vi "Versioned Load.vi"(10 "path":path) -> (0 "Reversals":T10, 1 "Trajectory Data":T1, 2 "Zero V":bool, 3 "Commands out":cluster{"Time (s)":dbl, T8, bool}[](array[cluster]), 4 "Fields":T7 {"Overrides"."Angle Override" step=5.0; "Overrides"."Velocity Override" step=5.0; "Overrides"."Angular Override" step=5.0; "Angular Limits"."Jerk (deg/s^3)" min=0.0 step=1.0; "Angular Limits"."Accel (deg/s^2)" min=0.0; "Angular Limits"."Velocity (deg/s)" min=0.0}, 5 "Points out":cluster{"x":dbl, "y":dbl, "th":dbl}[](array[cluster]), 6 "Trajectory Meta":cluster{"Drive Type":T3, "Path Type":T4}, 7 "Overall":cluster{"Time (s)":dbl, "Distance (ft)":dbl}, 8 "error out":errorcluster)   [LabVIEW 2023]
uses:
  Types/Single Cmd Info.ctl
  <vilib>/picture/picture.llb/imagedata.ctl
  Types/Overrides.ctl
  Types/Angluar Limits.ctl
  Types/Drive Type.ctl
  Types/Path Type.ctl
  Types/Trajectory Data.ctl
  Types/Segment Type.ctl
  Types/Availible Command systems for auto.ctl
  Types/Limits.ctl
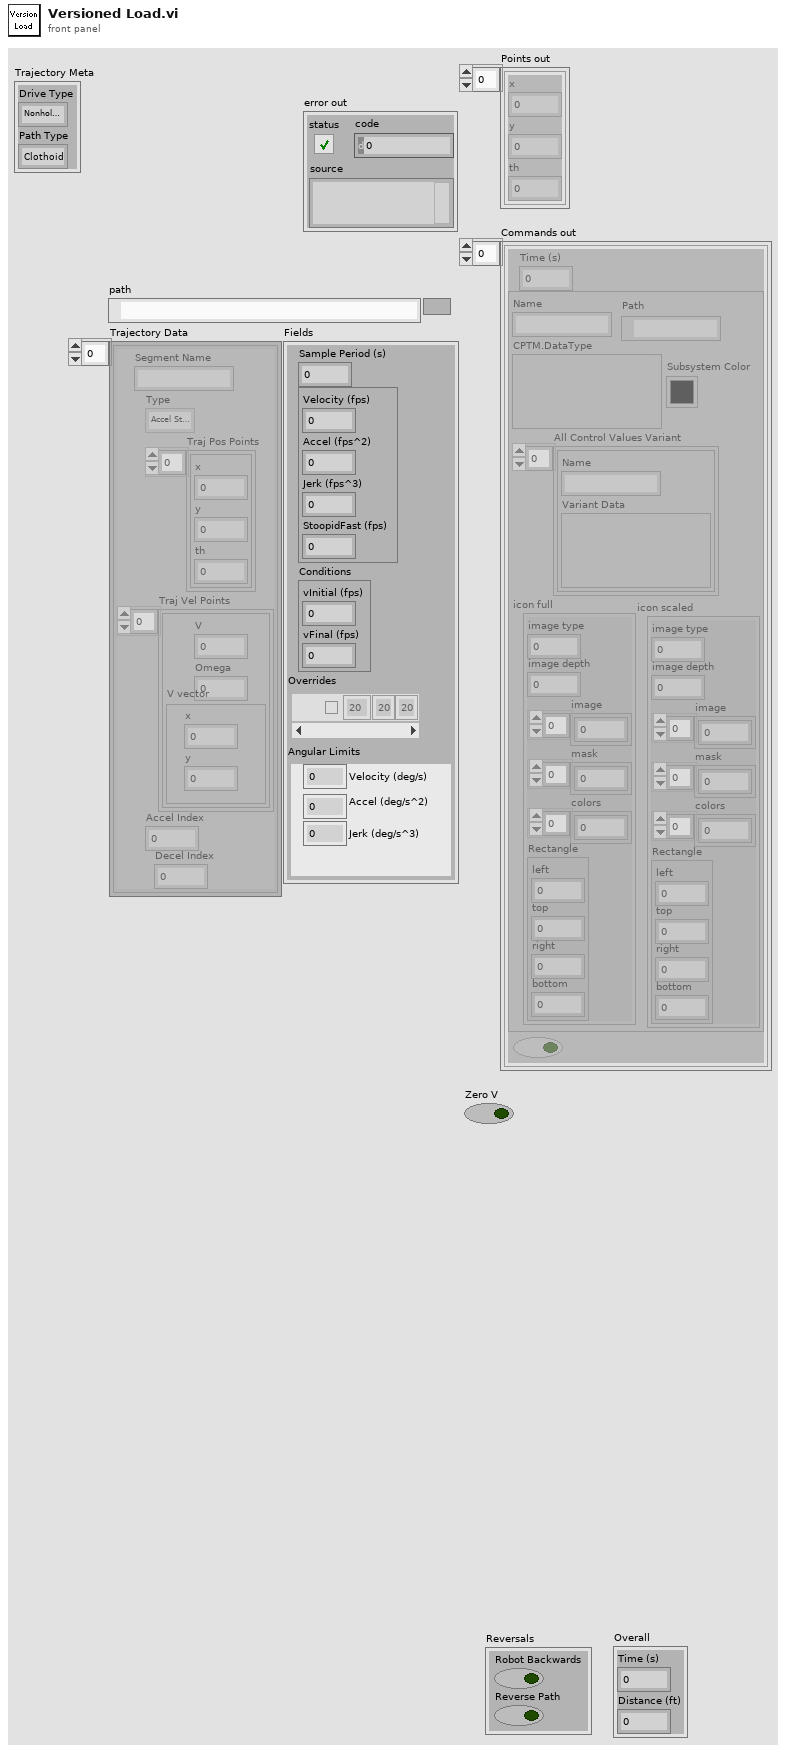
[diagram p1: front panel]
types:
  T1 = typedef "Trajectory Data.ctl" = cluster{"Segment Name":string, "Type":T2, "Traj Pos Points":cluster{"x":dbl, "y":dbl, "th":dbl}[], "Traj Vel Points":cluster{"V":dbl, "Omega":dbl, "V vector":cluster{"y":dbl, "x":dbl}}[], "Accel Index":i32, "Decel Index":i32}[]
  T2 = typedef "Segment Type.ctl" = enum16{"Accel Straight", "Const Straight", "Blend", "Circle", "Bezier"}
  T3 = typedef "Drive Type.ctl" = enum16{"Nonholonomic", "Holonomic"}
  T4 = typedef "Path Type.ctl" = enum16{"Clothoid", "Bezier"}
  T5 = typedef "Overrides.ctl" = cluster{"Count":string, "Angular Override":dbl, "Enabled?":bool, "Velocity Override":dbl, "Angle Override":dbl}[]
  T6 = typedef "Angluar Limits.ctl" = cluster{"Velocity (deg/s)":dbl, "Accel (deg/s^2)":dbl, "Jerk (deg/s^3)":dbl}
  T7 = cluster{"Sample Period (s)":dbl, cluster{"Velocity (fps)":dbl, "Accel (fps^2)":dbl, "Jerk (fps^3)":dbl, "StoopidFast (fps)":dbl}, "Conditions":cluster{"vInitial (fps)":dbl, "vFinal (fps)":dbl}, "Overrides":T5, "Angular Limits":T6}
  T8 = typedef "Single Cmd Info.ctl" = cluster{"Name":string, "CPTM.DataType":variant, "All Control Values Variant":cluster{"Name":string, "Variant Data":variant}[], "icon full":T9, "icon scaled":T9, "Path":path, "Subsystem Color":u32}
  T9 = typedef "imagedata.ctl" = cluster{"image type":i32, "image depth":i32, "image":u8[], "mask":u8[], "colors":u32[], "Rectangle":cluster{"left":i16, "top":i16, "right":i16, "bottom":i16}}
  T10 = cluster{"Robot Backwards":bool, "Reverse Path":bool}
  T11 = cluster{"Segment Name":string, "Type":T2, "Traj Pos Points":cluster{"x":dbl, "y":dbl, "th":dbl}[], "Traj Vel Points":cluster{"V":dbl, "Omega":dbl}[], "Accel Index":i32, "Decel Index":i32}[]
  T12 = cluster{"Sample Period (s)":dbl, "Limits 2":cluster{"Velocity (fps)":dbl, "Acceleration (fps^2)":dbl, "Jerk (fps^3)":dbl}, "Conditions":cluster{"vInitial (fps)":dbl, "vFinal (fps)":dbl}, " Acceleration Overrides":cluster{"Angular \nAccelerations":dbl[], "Accel Override Bools":bool[]}}
  T13 = cluster{"Velocity":dbl, "Sample Time":dbl, "Accel":dbl}
  T14 = cluster{"Sample Period (s)":dbl, "Limits":cluster{"Velocity (fps)":dbl, "Acceleration (fps^2)":dbl, "Jerk (fps^3)":dbl}, "Conditions":cluster{"vInitial (fps)":dbl, "vFinal (fps)":dbl}}
  T15 = cluster{"Sample Period (s)":dbl, "Limits":cluster{"Velocity (fps)":dbl, "Acceleration (fps^2)":dbl, "Jerk (fps^3)":dbl}, "Conditions":cluster{"vInitial (fps)":dbl, "vFinal (fps)":dbl}, "Min Rads":dbl[]}
  T16 = typedef "Availible Command systems for auto.ctl" = u16
  T17 = cluster{"Time into Path":dbl, "System":T16, "Item Selected?":bool, "System Selection":T16}[]
  T18 = cluster{"Sample Period (s)":dbl, "Limits 2":cluster{"Velocity (fps)":dbl, "Acceleration (fps^2)":dbl, "Jerk (fps^3)":dbl, "Stoopid Fast":dbl}, "Conditions":cluster{"vInitial (fps)":dbl, "vFinal (fps)":dbl}, " Acceleration Overrides":cluster{"Angular \nAccelerations":dbl[], "Accel Override Bools":bool[]}}
  T19 = cluster{"Sample Period (s)":dbl, "Limits":cluster{"Velocity (fps)":dbl, "Accel (fps^2)":dbl, "Turn Accel (fps^2)":dbl, "Jerk (fps^3)":dbl}, "Conditions":cluster{"vInitial (fps)":dbl, "vFinal (fps)":dbl}, cluster{dbl[], bool[]}}
  T20 = cluster{"Reverse Path":bool, "Robot Backwards":bool}
  T21 = typedef "Limits.ctl" = cluster{"Velocity (fps)":dbl, "Accel (fps^2)":dbl, "Jerk (fps^3)":dbl, "StoopidFast (fps)":dbl}
  T22 = cluster{"Sample Period (s)":dbl, "Limits":T21, "Conditions":cluster{"vInitial (fps)":dbl, "vFinal (fps)":dbl}, "Overrides":T5, "Angular Limits":T6}
  T23 = cluster{"Velocity":dbl, "Accel":dbl, "Accel":dbl, "Velocity":dbl}
  T24 = cluster{"Velocity (fps)":dbl, "Acceleration (fps^2)":dbl, "Jerk (fps^3)":dbl}
  T25 = cluster{"vInitial (fps)":dbl, "vFinal (fps)":dbl}
  T26 = cluster{"Velocity (fps)":dbl, "Acceleration (fps^2)":dbl, "Jerk (fps^3)":dbl, "Velocity (fps)":dbl}
  T27 = cluster{string, "Angular Multiplier":dbl, bool, "Velocity (fps)":dbl, "Velocity (fps)":dbl}
  T28 = cluster{"Angular \nAccelerations":dbl[], "Accel Override Bools":bool[]}
  T29 = cluster{"Velocity (fps)":dbl, "Acceleration (fps^2)":dbl, "Jerk (fps^3)":dbl, "Stoopid Fast":dbl}
  T30 = cluster{"Velocity (fps)":dbl, "Accel (fps^2)":dbl, "Turn Accel (fps^2)":dbl, "Jerk (fps^3)":dbl}
  T31 = cluster{"Velocity (fps)":dbl, "Accel (fps^2)":dbl, "Jerk (fps^3)":dbl, "StoopidFast (fps)":dbl}
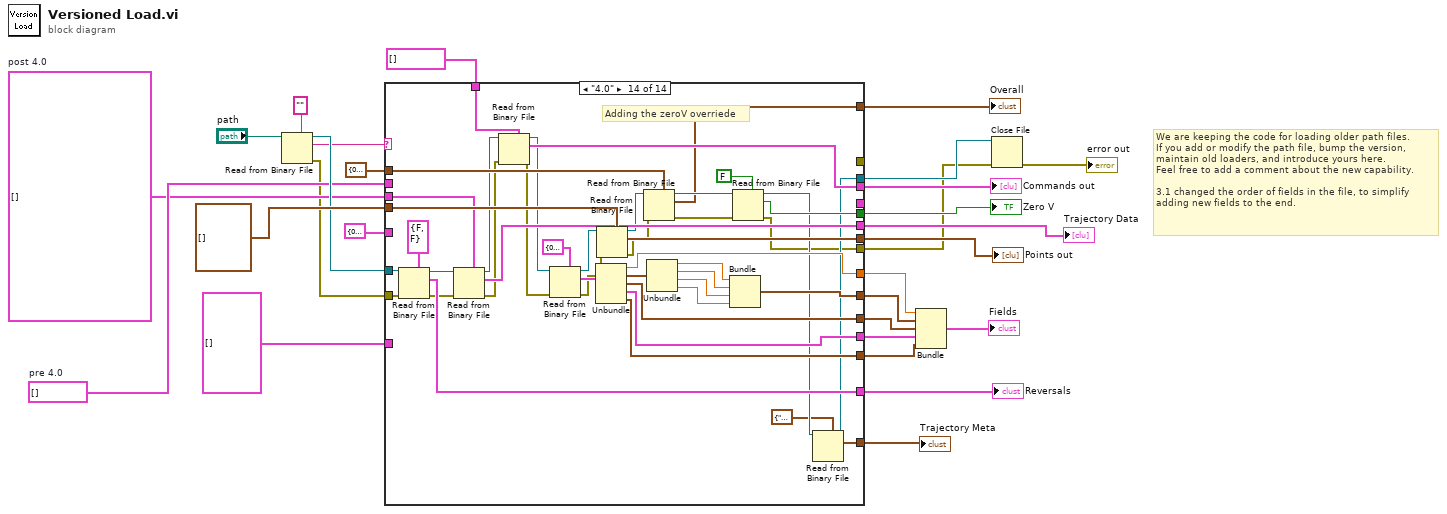
[diagram p0: block diagram]
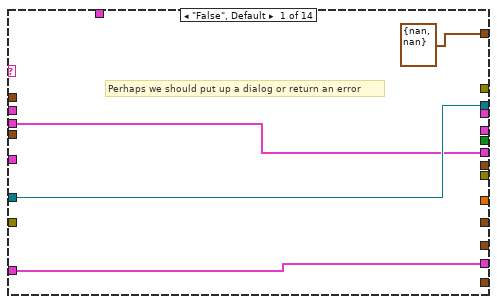
[diagram p2: hidden frame]
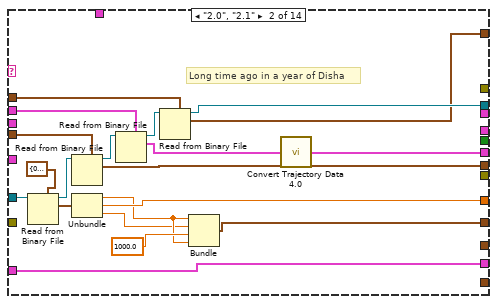
[diagram p3: hidden frame]
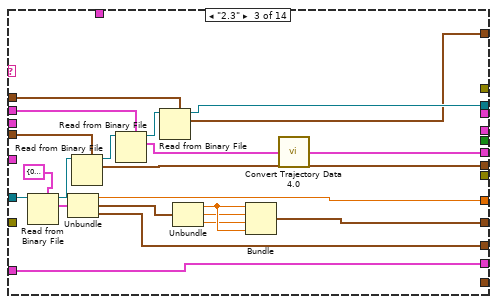
[diagram p4: hidden frame]
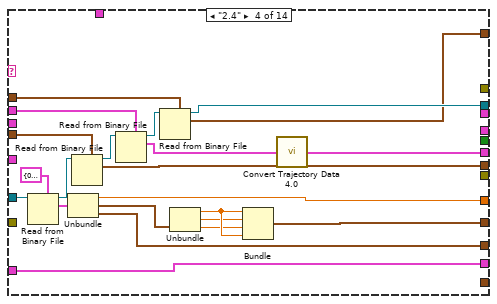
[diagram p5: hidden frame]
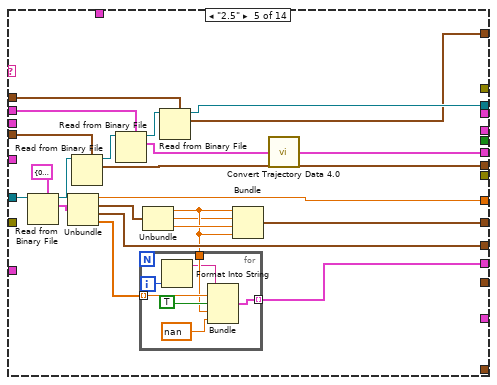
[diagram p6: hidden frame]
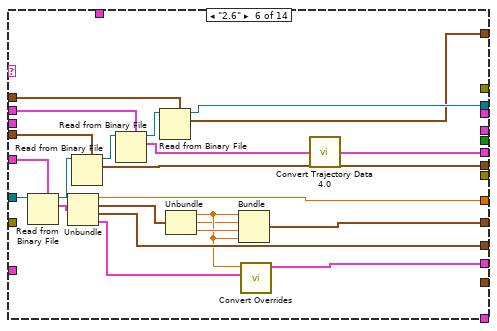
[diagram p7: hidden frame]
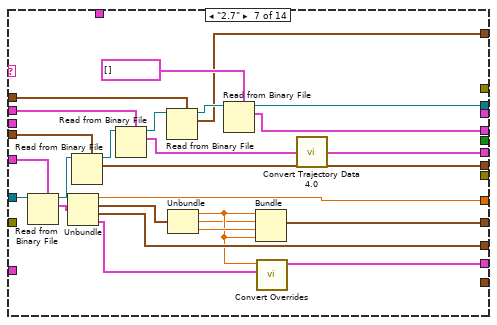
[diagram p8: hidden frame]
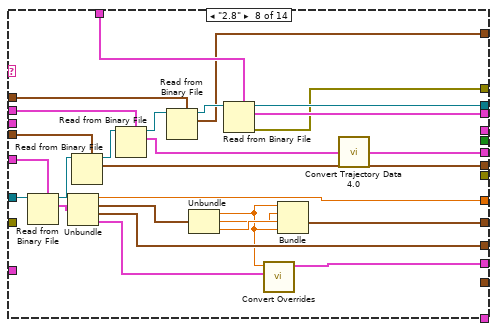
[diagram p9: hidden frame]
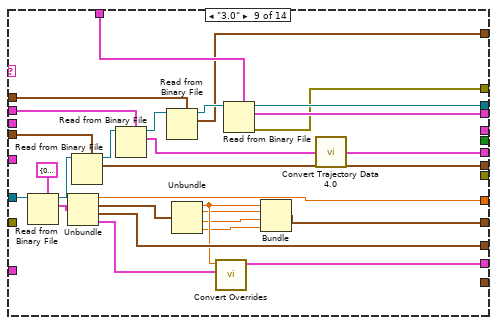
[diagram p10: hidden frame]
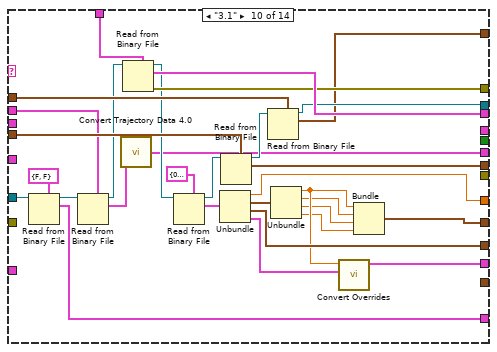
[diagram p11: hidden frame]
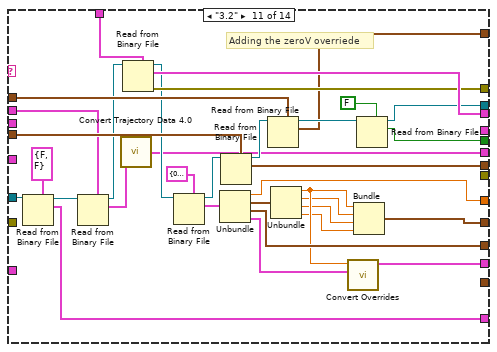
[diagram p12: hidden frame]
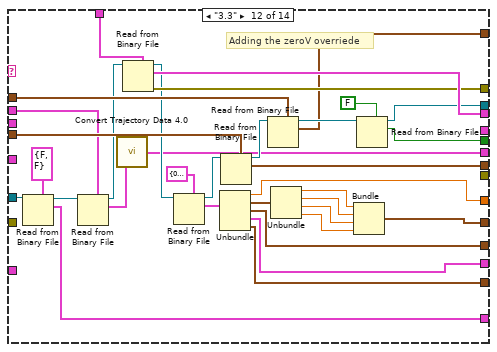
[diagram p13: hidden frame]
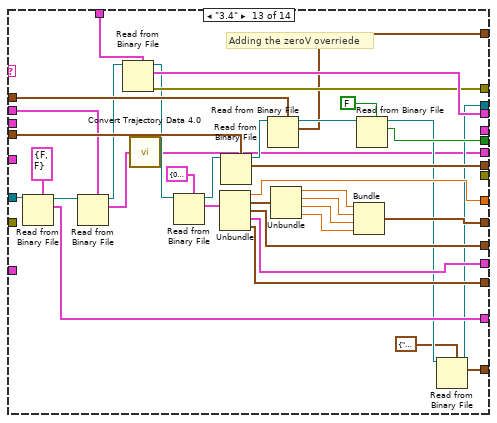
[diagram p14: hidden frame]
diagram:
  w6 = T11 []  # pre 4.0
  w5 = T1 []  # post 4.0
  # "We are keeping the code for loading older path files.\nIf you add or modify the path file, bump the version,\nmaintain old loaders, and introduce yours here.\nFeel free to add a comment about the new capability.\n\n3.1 changed the order of fields in the file, to simplify\nadding new fields to the end."
  n1 = Read from Binary File(5:"" ("String"), 11:"path") -> (0:w3:errorcluster, 2:w12:string, 3:w13:refnum<file>)  [unwired: 4 in, 1 out]
  n2 = case shown="\"4.0\"" w12 {
    tunnel: w13 -> [w32 w51 w73 w95 w118 w148 w174 w201 w229 w250 w284 w318 w355 w400]
    tunnel: cluster{"x":dbl, "y":dbl, "th":dbl}[] [] ("Points in") -> [_ w49 w71 w93 w116 w146 w172 w199 w227 w259 w293 w327 w364 w407]
    tunnel: [_ w48 w70 w92 w115 w145 w171 w198 w226 w258 w292 w326 w363 w406] -> w18
    tunnel: w6 -> [_ w47 w69 w91 w114 w144 w170 w197 w225 w257 w291 w325 w362 _]
    tunnel: cluster{"Time (s)":dbl, "Distance (ft)":dbl} {"Time (s)"=0.0, "Distance (ft)"=0.0} ("Cluster 4") -> [_ w45 w67 w89 w112 w142 w168 w195 w223 w256 w290 w324 w361 w405]
    tunnel: [w32 w43 w65 w87 w110 w140 w162 w189 w217 w246 w266 w303 w332 w377] -> w15
    tunnel: [_ w41 w64 w86 w109 w139 w166 w193 w221 w233 w268 w305 w342 w387] -> w25
    tunnel: [_ w37 w58 w79 w103 w134 w156 w184 w205 w238 w273 w310 w347 w392] -> w26
    tunnel: [_ _ w63 w85 w108 w138 w165 w192 w220 w255 w289 w323 w360 w404] -> w27
    tunnel: [w31 w36 w57 w78 w102 w132 w153 w181 w211 w242 w277 w298 w336 w381] -> w28
    tunnel: [w29 w33 w53 w75 w97 w127 w150 w176 w203 w231 w262 w296 w330 w403] -> w4
    tunnel: [_ _ _ _ _ _ w161 _ _ _ _ _ _ _] -> _
    tunnel: cluster{"Time (s)":dbl, T8, bool}[] [] ("Commands in") -> [_ _ _ _ _ _ _ w188 w216 w253 w287 w321 w358 w402]
    tunnel: [_ _ _ _ _ _ _ w187 w215 w252 w286 w320 w357 w401] -> w20
    tunnel: [_ _ _ _ _ _ _ w186 w214 w251 w285 w319 w356 _] -> _
    tunnel: T12 {"Sample Period (s)"=0.0, "Limits 2"={"Velocity (fps)"=0.0, "Acceleration (fps^2)"=0.0, "Jerk (fps^3)"=0.0}, "Conditions"={"vInitial (fps)"=0.0, "vFinal (fps)"=0.0}, " Acceleration Overrides"={"Angular \nAccelerations"=[], "Accel Override Bools"=[]}} ("Cluster") -> [_ _ _ _ _ w136 w159 w182 _ _ _ _ _ _]
    tunnel: [_ _ _ _ _ _ _ _ _ w241 w276 w312 w349 w394] -> w22
    tunnel: T5 [] ("Overrides") -> [w31 w36 w57 w78 _ _ _ _ _ _ _ _ _ _]
    tunnel: [_ _ _ _ _ _ _ _ _ _ w264 w301 w339 w384] -> w23
    tunnel: [cluster{"Time (s)":dbl, "Distance (ft)":dbl} {"Time (s)"=nan, "Distance (ft)"=nan} ("Cluster 4") w34 w54 w76 w98 w128 w151 w177 w204 w232 w263 w300 w338 w383] -> w10
    tunnel: [_ _ _ _ _ _ _ _ _ _ _ w297 w335 w380] -> w8
    tunnel: [_ _ _ _ _ _ _ _ _ _ _ _ w331 w376] -> w7
    tunnel: w5 -> [w29 _ _ _ _ _ _ _ _ _ _ _ _ w375]
    tunnel: w3 -> [_ _ _ _ _ _ _ _ _ _ _ _ _ w373]
    tunnel: [_ _ _ _ _ _ _ _ _ _ _ _ _ w367] -> w1
    frame "False", Default {
      # "Perhaps we should put up a dialog or return an error"
    }
    frame "2.0", "2.1" {
      # "Long time ago in a year of Disha"
      n3 = Read from Binary File(5:T13 {"Velocity"=0.0, "Sample Time"=0.0, "Accel"=0.0}, 11:w51) -> (2:w52:T13, 3:w50:refnum<file>)  [unwired: 4 in, 2 out]
      n4 = Read from Binary File(5:w49, 11:w50) -> (2:w48:cluster{"x":dbl, "y":dbl, "th":dbl}[], 3:w46:refnum<file>)  [unwired: 4 in, 2 out]
      n5 = Unbundle(w52) -> ("Velocity"=w38:dbl, "Sample Time"=w41:dbl, "Accel"=w35:dbl)
      n6 = Read from Binary File(5:w47, 11:w46) -> (2:w39:T11, 3:w44:refnum<file>)  [unwired: 4 in, 2 out]
      n7 = Read from Binary File(5:w45, 11:w44) -> (2:w34:cluster{"Time (s)":dbl, "Distance (ft)":dbl}, 3:w43:refnum<file>)  [unwired: 4 in, 2 out]
      n8 = Bundle("Velocity"=w38, "Accel"=w35, "Accel"=1000.0, "Velocity"=w38) -> (w37:T23)  [unwired: 1 in]
      n9 = call "Convert Trajectory Data 4.0.vi"("pre 4.0"=w39) -> ("post 4.0"=w33:T1)
    }
    frame "2.3" {
      n10 = Read from Binary File(5:T14 {"Sample Period (s)"=0.0, "Limits"={"Velocity (fps)"=0.0, "Acceleration (fps^2)"=0.0, "Jerk (fps^3)"=0.0}, "Conditions"={"vInitial (fps)"=0.0, "vFinal (fps)"=0.0}}, 11:w73) -> (2:w74:T14, 3:w72:refnum<file>)  [unwired: 4 in, 2 out]
      n11 = Unbundle(w74) -> ("Sample Period (s)"=w64:dbl, "Limits"=w55:T24, "Conditions"=w63:T25)
      n12 = Read from Binary File(5:w71, 11:w72) -> (2:w70:cluster{"x":dbl, "y":dbl, "th":dbl}[], 3:w68:refnum<file>)  [unwired: 4 in, 2 out]
      n13 = Read from Binary File(5:w69, 11:w68) -> (2:w61:T11, 3:w66:refnum<file>)  [unwired: 4 in, 2 out]
      n14 = Read from Binary File(5:w67, 11:w66) -> (2:w54:cluster{"Time (s)":dbl, "Distance (ft)":dbl}, 3:w65:refnum<file>)  [unwired: 4 in, 2 out]
      n15 = Unbundle(w55) -> ("Velocity (fps)"=w60:dbl, "Acceleration (fps^2)"=w56:dbl, "Jerk (fps^3)"=w59:dbl)
      n16 = Bundle("Velocity (fps)"=w60, "Acceleration (fps^2)"=w56, "Jerk (fps^3)"=w59, "Velocity (fps)"=w60) -> (w58:T26)  [unwired: 1 in]
      n17 = call "Convert Trajectory Data 4.0.vi"("pre 4.0"=w61) -> ("post 4.0"=w53:T1)
    }
    frame "2.4" {
      n18 = Read from Binary File(5:T14 {"Sample Period (s)"=0.0, "Limits"={"Velocity (fps)"=0.0, "Acceleration (fps^2)"=0.0, "Jerk (fps^3)"=0.0}, "Conditions"={"vInitial (fps)"=0.0, "vFinal (fps)"=0.0}}, 11:w95) -> (2:w96:T14, 3:w94:refnum<file>)  [unwired: 4 in, 2 out]
      n19 = Unbundle(w96) -> ("Sample Period (s)"=w86:dbl, "Limits"=w80:T24, "Conditions"=w85:T25)
      n20 = Read from Binary File(5:w93, 11:w94) -> (2:w92:cluster{"x":dbl, "y":dbl, "th":dbl}[], 3:w90:refnum<file>)  [unwired: 4 in, 2 out]
      n21 = Read from Binary File(5:w91, 11:w90) -> (2:w83:T11, 3:w88:refnum<file>)  [unwired: 4 in, 2 out]
      n22 = Read from Binary File(5:w89, 11:w88) -> (2:w76:cluster{"Time (s)":dbl, "Distance (ft)":dbl}, 3:w87:refnum<file>)  [unwired: 4 in, 2 out]
      n23 = Unbundle(w80) -> ("Velocity (fps)"=w82:dbl, "Acceleration (fps^2)"=w77:dbl, "Jerk (fps^3)"=w81:dbl)
      n24 = Bundle("Velocity (fps)"=w82, "Acceleration (fps^2)"=w77, "Jerk (fps^3)"=w81, "Velocity (fps)"=w82) -> (w79:T26)  [unwired: 1 in]
      n25 = call "Convert Trajectory Data 4.0.vi"("pre 4.0"=w83) -> ("post 4.0"=w75:T1)
    }
    frame "2.5" {
      n26 = Read from Binary File(5:T15 {"Sample Period (s)"=0.0, "Limits"={"Velocity (fps)"=0.0, "Acceleration (fps^2)"=0.0, "Jerk (fps^3)"=0.0}, "Conditions"={"vInitial (fps)"=0.0, "vFinal (fps)"=0.0}, "Min Rads"=[20.0, 20.0, 20.0, 20.0, 20.0]}, 11:w118) -> (2:w119:T15, 3:w117:refnum<file>)  [unwired: 4 in, 2 out]
      n27 = Unbundle(w119) -> ("Sample Period (s)"=w109:dbl, "Limits"=w104:T24, "Conditions"=w108:T25, "Min Rads"=w101:dbl[])
      n28 = Read from Binary File(5:w116, 11:w117) -> (2:w115:cluster{"x":dbl, "y":dbl, "th":dbl}[], 3:w113:refnum<file>)  [unwired: 4 in, 2 out]
      n29 = Read from Binary File(5:w114, 11:w113) -> (2:w106:T11, 3:w111:refnum<file>)  [unwired: 4 in, 2 out]
      n30 = Unbundle(w104) -> ("Velocity (fps)"=w100:dbl, "Acceleration (fps^2)"=w99:dbl, "Jerk (fps^3)"=w105:dbl)
      n31 = for {
        tunnel: [w125] -> w102 mode=indexing
        tunnel: w101 -> [w124] mode=indexing
        tunnel: w100 -> [w123]
        i -> [w122]
        n32 = Format Into String(w122) -> (resulting string=w121:string)  [unwired: 3 in, 1 out]
        n33 = Bundle(w121, "Angular Multiplier"=w124, TRUE, "Velocity (fps)"=w123, "Velocity (fps)"=nan) -> (w125:T27)  [unwired: 1 in]
      }
      n34 = Read from Binary File(5:w112, 11:w111) -> (2:w98:cluster{"Time (s)":dbl, "Distance (ft)":dbl}, 3:w110:refnum<file>)  [unwired: 4 in, 2 out]
      n35 = Bundle("Velocity (fps)"=w100, "Acceleration (fps^2)"=w99, "Jerk (fps^3)"=w105, "Velocity (fps)"=w100) -> (w103:T26)  [unwired: 1 in]
      n36 = call "Convert Trajectory Data 4.0.vi"("pre 4.0"=w106) -> ("post 4.0"=w97:T1)
    }
    frame "2.6" {
      n37 = Read from Binary File(5:w136, 11:w148) -> (2:w149:T12, 3:w147:refnum<file>)  [unwired: 4 in, 2 out]
      n38 = Unbundle(w149) -> ("Sample Period (s)"=w139:dbl, "Limits 2"=w133:T24, "Conditions"=w138:T25, "Acceleration Overrides"=w130:T28)
      n39 = Read from Binary File(5:w146, 11:w147) -> (2:w145:cluster{"x":dbl, "y":dbl, "th":dbl}[], 3:w143:refnum<file>)  [unwired: 4 in, 2 out]
      n40 = Read from Binary File(5:w144, 11:w143) -> (2:w137:T11, 3:w141:refnum<file>)  [unwired: 4 in, 2 out]
      n41 = Read from Binary File(5:w142, 11:w141) -> (2:w128:cluster{"Time (s)":dbl, "Distance (ft)":dbl}, 3:w140:refnum<file>)  [unwired: 4 in, 2 out]
      n42 = Unbundle(w133) -> ("Velocity (fps)"=w131:dbl, "Acceleration (fps^2)"=w129:dbl, "Jerk (fps^3)"=w135:dbl)
      n43 = Bundle("Velocity (fps)"=w131, "Acceleration (fps^2)"=w129, "Jerk (fps^3)"=w135, "Velocity (fps)"=w131) -> (w134:T26)  [unwired: 1 in]
      n44 = call "Convert Overrides.vi"("Cluster"=w130, "Velocity (fps)"=w131) -> ("Overrides"=w132:T5)  [unwired: 9 in]
      n45 = call "Convert Trajectory Data 4.0.vi"("pre 4.0"=w137) -> ("post 4.0"=w127:T1)
    }
    frame "2.7" {
      n46 = Read from Binary File(5:w159, 11:w174) -> (2:w175:T12, 3:w173:refnum<file>)  [unwired: 4 in, 2 out]
      n47 = Unbundle(w175) -> ("Sample Period (s)"=w166:dbl, "Limits 2"=w157:T24, "Conditions"=w165:T25, "Acceleration Overrides"=w154:T28)
      n48 = Read from Binary File(5:w172, 11:w173) -> (2:w171:cluster{"x":dbl, "y":dbl, "th":dbl}[], 3:w169:refnum<file>)  [unwired: 4 in, 2 out]
      n49 = Read from Binary File(5:w170, 11:w169) -> (2:w164:T11, 3:w167:refnum<file>)  [unwired: 4 in, 2 out]
      n50 = Read from Binary File(5:w168, 11:w167) -> (2:w151:cluster{"Time (s)":dbl, "Distance (ft)":dbl}, 3:w163:refnum<file>)  [unwired: 4 in, 2 out]
      n51 = Unbundle(w157) -> ("Velocity (fps)"=w155:dbl, "Acceleration (fps^2)"=w152:dbl, "Jerk (fps^3)"=w158:dbl)
      n52 = Read from Binary File(5:T17 [] ("Commands"), 11:w163) -> (2:w161:T17, 3:w162:refnum<file>)  [unwired: 4 in, 2 out]
      n53 = Bundle("Velocity (fps)"=w155, "Acceleration (fps^2)"=w152, "Jerk (fps^3)"=w158, "Velocity (fps)"=w155) -> (w156:T26)  [unwired: 1 in]
      n54 = call "Convert Overrides.vi"("Cluster"=w154, "Velocity (fps)"=w155) -> ("Overrides"=w153:T5)  [unwired: 9 in]
      n55 = call "Convert Trajectory Data 4.0.vi"("pre 4.0"=w164) -> ("post 4.0"=w150:T1)
    }
    frame "2.8" {
      n56 = Read from Binary File(5:w182, 11:w201) -> (2:w202:T12, 3:w200:refnum<file>)  [unwired: 4 in, 2 out]
      n57 = Unbundle(w202) -> ("Sample Period (s)"=w193:dbl, "Limits 2"=w185:T24, "Conditions"=w192:T25, "Acceleration Overrides"=w179:T28)
      n58 = Read from Binary File(5:w199, 11:w200) -> (2:w198:cluster{"x":dbl, "y":dbl, "th":dbl}[], 3:w196:refnum<file>)  [unwired: 4 in, 2 out]
      n59 = Read from Binary File(5:w197, 11:w196) -> (2:w191:T11, 3:w194:refnum<file>)  [unwired: 4 in, 2 out]
      n60 = Read from Binary File(5:w195, 11:w194) -> (2:w177:cluster{"Time (s)":dbl, "Distance (ft)":dbl}, 3:w190:refnum<file>)  [unwired: 4 in, 2 out]
      n61 = Unbundle(w185) -> ("Velocity (fps)"=w180:dbl, "Acceleration (fps^2)"=w178:dbl, "Jerk (fps^3)"=w183:dbl)
      n62 = Read from Binary File(5:w188, 11:w190) -> (0:w186:errorcluster, 2:w187:cluster{"Time (s)":dbl, T8, bool}[], 3:w189:refnum<file>)  [unwired: 4 in, 1 out]
      n63 = call "Convert Overrides.vi"("Cluster"=w179, "Velocity (fps)"=w180) -> ("Overrides"=w181:T5)  [unwired: 9 in]
      n64 = Bundle("Velocity (fps)"=w180, "Acceleration (fps^2)"=w178, "Jerk (fps^3)"=w183, "Velocity (fps)"=w180) -> (w184:T26)  [unwired: 1 in]
      n65 = call "Convert Trajectory Data 4.0.vi"("pre 4.0"=w191) -> ("post 4.0"=w176:T1)
    }
    frame "3.0" {
      n66 = Read from Binary File(5:T18 {"Sample Period (s)"=0.0, "Limits 2"={"Velocity (fps)"=0.0, "Acceleration (fps^2)"=0.0, "Jerk (fps^3)"=0.0, "Stoopid Fast"=0.0}, "Conditions"={"vInitial (fps)"=0.0, "vFinal (fps)"=0.0}, " Acceleration Overrides"={"Angular \nAccelerations"=[], "Accel Override Bools"=[]}} ("Cluster"), 11:w229) -> (2:w230:T18, 3:w228:refnum<file>)  [unwired: 4 in, 2 out]
      n67 = Unbundle(w230) -> ("Sample Period (s)"=w221:dbl, "Limits 2"=w206:T29, "Conditions"=w220:T25, "Acceleration Overrides"=w212:T28)
      n68 = Read from Binary File(5:w227, 11:w228) -> (2:w226:cluster{"x":dbl, "y":dbl, "th":dbl}[], 3:w224:refnum<file>)  [unwired: 4 in, 2 out]
      n69 = Read from Binary File(5:w225, 11:w224) -> (2:w219:T11, 3:w222:refnum<file>)  [unwired: 4 in, 2 out]
      n70 = Read from Binary File(5:w223, 11:w222) -> (2:w204:cluster{"Time (s)":dbl, "Distance (ft)":dbl}, 3:w218:refnum<file>)  [unwired: 4 in, 2 out]
      n71 = Unbundle(w206) -> ("Velocity (fps)"=w210:dbl, "Acceleration (fps^2)"=w209:dbl, "Jerk (fps^3)"=w208:dbl, "Stoopid Fast"=w207:dbl)
      n72 = call "Convert Overrides.vi"("Cluster"=w212, "Velocity (fps)"=w210) -> ("Overrides"=w211:T5)  [unwired: 9 in]
      n73 = Read from Binary File(5:w216, 11:w218) -> (0:w214:errorcluster, 2:w215:cluster{"Time (s)":dbl, T8, bool}[], 3:w217:refnum<file>)  [unwired: 4 in, 1 out]
      n74 = Bundle("Velocity (fps)"=w210, "Acceleration (fps^2)"=w209, "Jerk (fps^3)"=w208, "Stoopid Fast"=w207) -> (w205:T29)  [unwired: 1 in]
      n75 = call "Convert Trajectory Data 4.0.vi"("pre 4.0"=w219) -> ("post 4.0"=w203:T1)
    }
    frame "3.1" {
      n76 = Read from Binary File(5:T20 {"Reverse Path"=FALSE, "Robot Backwards"=FALSE} ("Cluster"), 11:w250) -> (2:w241:T20, 3:w247:refnum<file>)  [unwired: 4 in, 2 out]
      n77 = Read from Binary File(5:w257, 11:w247) -> (2:w254:T11, 3:w245:refnum<file>)  [unwired: 4 in, 2 out]
      n78 = call "Convert Trajectory Data 4.0.vi"("pre 4.0"=w254) -> ("post 4.0"=w231:T1)
      n79 = Read from Binary File(5:w253, 11:w245) -> (0:w251:errorcluster, 2:w252:cluster{"Time (s)":dbl, T8, bool}[], 3:w244:refnum<file>)  [unwired: 4 in, 1 out]
      n80 = Read from Binary File(5:T19 {"Sample Period (s)"=0.0, "Limits"={"Velocity (fps)"=0.0, "Accel (fps^2)"=0.0, "Turn Accel (fps^2)"=15.0, "Jerk (fps^3)"=0.0}, "Conditions"={"vInitial (fps)"=0.0, "vFinal (fps)"=0.0}, {[], []}} ("Cluster 2"), 11:w244) -> (2:w261:T19, 3:w260:refnum<file>)  [unwired: 4 in, 2 out]
      n81 = Unbundle(w261) -> ("Sample Period (s)"=w233:dbl, "Limits"=w240:T30, "Conditions"=w255:T25, w243:cluster{dbl[], bool[]})
      n82 = Read from Binary File(5:w259, 11:w260) -> (2:w258:cluster{"x":dbl, "y":dbl, "th":dbl}[], 3:w248:refnum<file>)  [unwired: 4 in, 2 out]
      n83 = Read from Binary File(5:w256, 11:w248) -> (2:w232:cluster{"Time (s)":dbl, "Distance (ft)":dbl}, 3:w246:refnum<file>)  [unwired: 4 in, 2 out]
      n84 = Unbundle(w240) -> ("Velocity (fps)"=w237:dbl, "Accel (fps^2)"=w236:dbl, "Turn Accel (fps^2)"=w235:dbl, "Jerk (fps^3)"=w234:dbl)
      n85 = call "Convert Overrides.vi"("Cluster"=w243, "Velocity (fps)"=w237) -> ("Overrides"=w242:T5)  [unwired: 9 in]
      n86 = Bundle("Velocity (fps)"=w237, "Accel (fps^2)"=w236, "Turn Accel (fps^2)"=w235, "Jerk (fps^3)"=w234) -> (w238:T30)  [unwired: 1 in]
    }
    frame "3.2" {
      # "Adding the zeroV overriede"
      n87 = Read from Binary File(5:T10 {"Robot Backwards"=FALSE, "Reverse Path"=FALSE} ("Cluster"), 11:w284) -> (2:w276:T10, 3:w281:refnum<file>)  [unwired: 4 in, 2 out]
      n88 = Read from Binary File(5:w291, 11:w281) -> (2:w288:T11, 3:w280:refnum<file>)  [unwired: 4 in, 2 out]
      n89 = call "Convert Trajectory Data 4.0.vi"("pre 4.0"=w288) -> ("post 4.0"=w262:T1)
      n90 = Read from Binary File(5:w287, 11:w280) -> (0:w285:errorcluster, 2:w286:cluster{"Time (s)":dbl, T8, bool}[], 3:w279:refnum<file>)  [unwired: 4 in, 1 out]
      n91 = Read from Binary File(5:T19 {"Sample Period (s)"=0.0, "Limits"={"Velocity (fps)"=0.0, "Accel (fps^2)"=0.0, "Turn Accel (fps^2)"=15.0, "Jerk (fps^3)"=0.0}, "Conditions"={"vInitial (fps)"=0.0, "vFinal (fps)"=0.0}, {[], []}} ("Cluster 2"), 11:w279) -> (2:w295:T19, 3:w294:refnum<file>)  [unwired: 4 in, 2 out]
      n92 = Unbundle(w295) -> ("Sample Period (s)"=w268:dbl, "Limits"=w275:T30, "Conditions"=w289:T25, w278:cluster{dbl[], bool[]})
      n93 = Read from Binary File(5:w293, 11:w294) -> (2:w292:cluster{"x":dbl, "y":dbl, "th":dbl}[], 3:w282:refnum<file>)  [unwired: 4 in, 2 out]
      n94 = Read from Binary File(5:w290, 11:w282) -> (2:w263:cluster{"Time (s)":dbl, "Distance (ft)":dbl}, 3:w267:refnum<file>)  [unwired: 4 in, 2 out]
      n95 = Unbundle(w275) -> ("Velocity (fps)"=w272:dbl, "Accel (fps^2)"=w271:dbl, "Turn Accel (fps^2)"=w270:dbl, "Jerk (fps^3)"=w269:dbl)
      n96 = call "Convert Overrides.vi"("Cluster"=w278, "Velocity (fps)"=w272) -> ("Overrides"=w277:T5)  [unwired: 9 in]
      n97 = Bundle("Velocity (fps)"=w272, "Accel (fps^2)"=w271, "Turn Accel (fps^2)"=w270, "Jerk (fps^3)"=w269) -> (w273:T30)  [unwired: 1 in]
      n98 = Read from Binary File(5:FALSE, 11:w267) -> (2:w264:bool, 3:w266:refnum<file>)  [unwired: 4 in, 2 out]
    }
    frame "3.3" {
      # "Adding the zeroV overriede"
      n99 = Read from Binary File(5:T10 {"Robot Backwards"=FALSE, "Reverse Path"=FALSE} ("Cluster"), 11:w318) -> (2:w312:T10, 3:w315:refnum<file>)  [unwired: 4 in, 2 out]
      n100 = Read from Binary File(5:w325, 11:w315) -> (2:w322:T11, 3:w314:refnum<file>)  [unwired: 4 in, 2 out]
      n101 = call "Convert Trajectory Data 4.0.vi"("pre 4.0"=w322) -> ("post 4.0"=w296:T1)
      n102 = Read from Binary File(5:w321, 11:w314) -> (0:w319:errorcluster, 2:w320:cluster{"Time (s)":dbl, T8, bool}[], 3:w313:refnum<file>)  [unwired: 4 in, 1 out]
      n103 = Read from Binary File(5:T22 {"Sample Period (s)"=0.0, "Limits"={"Velocity (fps)"=0.0, "Accel (fps^2)"=0.0, "Jerk (fps^3)"=0.0, "StoopidFast (fps)"=0.0}, "Conditions"={"vInitial (fps)"=0.0, "vFinal (fps)"=0.0}, "Overrides"=[], "Angular Limits"={"Velocity (deg/s)"=0.0, "Accel (deg/s^2)"=0.0, "Jerk (deg/s^3)"=0.0}} ("output cluster"), 11:w313) -> (2:w329:T22, 3:w328:refnum<file>)  [unwired: 4 in, 2 out]
      n104 = Unbundle(w329) -> ("Sample Period (s)"=w305:dbl, "Limits"=w311:T21, "Conditions"=w323:T25, "Overrides"=w298:T5, "Angular Limits"=w297:T6)
      n105 = Read from Binary File(5:w327, 11:w328) -> (2:w326:cluster{"x":dbl, "y":dbl, "th":dbl}[], 3:w316:refnum<file>)  [unwired: 4 in, 2 out]
      n106 = Read from Binary File(5:w324, 11:w316) -> (2:w300:cluster{"Time (s)":dbl, "Distance (ft)":dbl}, 3:w304:refnum<file>)  [unwired: 4 in, 2 out]
      n107 = Unbundle(w311) -> ("Velocity (fps)"=w309:dbl, "Accel (fps^2)"=w308:dbl, "Jerk (fps^3)"=w307:dbl, "StoopidFast (fps)"=w306:dbl)
      n108 = Bundle("Velocity (fps)"=w309, "Accel (fps^2)"=w308, "Jerk (fps^3)"=w307, "StoopidFast (fps)"=w306) -> (w310:T31)  [unwired: 1 in]
      n109 = Read from Binary File(5:FALSE, 11:w304) -> (2:w301:bool, 3:w303:refnum<file>)  [unwired: 4 in, 2 out]
    }
    frame "3.4" {
      # "Adding the zeroV overriede"
      n110 = Read from Binary File(5:T10 {"Robot Backwards"=FALSE, "Reverse Path"=FALSE} ("Cluster"), 11:w355) -> (2:w349:T10, 3:w352:refnum<file>)  [unwired: 4 in, 2 out]
      n111 = Read from Binary File(5:w362, 11:w352) -> (2:w359:T11, 3:w351:refnum<file>)  [unwired: 4 in, 2 out]
      n112 = Read from Binary File(5:w358, 11:w351) -> (0:w356:errorcluster, 2:w357:cluster{"Time (s)":dbl, T8, bool}[], 3:w350:refnum<file>)  [unwired: 4 in, 1 out]
      n113 = call "Convert Trajectory Data 4.0.vi"("pre 4.0"=w359) -> ("post 4.0"=w330:T1)
      n114 = Read from Binary File(5:T22 {"Sample Period (s)"=0.0, "Limits"={"Velocity (fps)"=0.0, "Accel (fps^2)"=0.0, "Jerk (fps^3)"=0.0, "StoopidFast (fps)"=0.0}, "Conditions"={"vInitial (fps)"=0.0, "vFinal (fps)"=0.0}, "Overrides"=[], "Angular Limits"={"Velocity (deg/s)"=0.0, "Accel (deg/s^2)"=0.0, "Jerk (deg/s^3)"=0.0}} ("output cluster"), 11:w350) -> (2:w366:T22, 3:w365:refnum<file>)  [unwired: 4 in, 2 out]
      n115 = Unbundle(w366) -> ("Sample Period (s)"=w342:dbl, "Limits"=w348:T21, "Conditions"=w360:T25, "Overrides"=w336:T5, "Angular Limits"=w335:T6)
      n116 = Read from Binary File(5:w364, 11:w365) -> (2:w363:cluster{"x":dbl, "y":dbl, "th":dbl}[], 3:w353:refnum<file>)  [unwired: 4 in, 2 out]
      n117 = Read from Binary File(5:w361, 11:w353) -> (2:w338:cluster{"Time (s)":dbl, "Distance (ft)":dbl}, 3:w341:refnum<file>)  [unwired: 4 in, 2 out]
      n118 = Unbundle(w348) -> ("Velocity (fps)"=w346:dbl, "Accel (fps^2)"=w345:dbl, "Jerk (fps^3)"=w344:dbl, "StoopidFast (fps)"=w343:dbl)
      n119 = Bundle("Velocity (fps)"=w346, "Accel (fps^2)"=w345, "Jerk (fps^3)"=w344, "StoopidFast (fps)"=w343) -> (w347:T31)  [unwired: 1 in]
      n120 = Read from Binary File(5:FALSE, 11:w341) -> (2:w339:bool, 3:w334:refnum<file>)  [unwired: 4 in, 2 out]
      n121 = Read from Binary File(5:cluster{"Drive Type":T3, "Path Type":T4} {"Drive Type"=enum."Nonholonomic", "Path Type"=enum."Clothoid"} ("Trajectory Meta"), 11:w334) -> (2:w331:cluster{"Drive Type":T3, "Path Type":T4}, 3:w332:refnum<file>)  [unwired: 4 in, 2 out]
    }
    frame "4.0" {
      # "Adding the zeroV overriede"
      n122 = Read from Binary File(5:T10 {"Robot Backwards"=FALSE, "Reverse Path"=FALSE} ("Cluster"), 8:w373, 11:w400) -> (0:w374:errorcluster, 2:w394:T10, 3:w397:refnum<file>)  [unwired: 3 in, 1 out]
      n123 = Read from Binary File(5:w375, 8:w374, 11:w397) -> (0:w372:errorcluster, 2:w403:T1, 3:w396:refnum<file>)  [unwired: 3 in, 1 out]
      n124 = Read from Binary File(5:w402, 8:w372, 11:w396) -> (0:w371:errorcluster, 2:w401:cluster{"Time (s)":dbl, T8, bool}[], 3:w395:refnum<file>)  [unwired: 3 in, 1 out]
      n125 = Read from Binary File(5:T22 {"Sample Period (s)"=0.0, "Limits"={"Velocity (fps)"=0.0, "Accel (fps^2)"=0.0, "Jerk (fps^3)"=0.0, "StoopidFast (fps)"=0.0}, "Conditions"={"vInitial (fps)"=0.0, "vFinal (fps)"=0.0}, "Overrides"=[], "Angular Limits"={"Velocity (deg/s)"=0.0, "Accel (deg/s^2)"=0.0, "Jerk (deg/s^3)"=0.0}} ("output cluster"), 8:w371, 11:w395) -> (0:w370:errorcluster, 2:w409:T22, 3:w408:refnum<file>)  [unwired: 3 in, 1 out]
      n126 = Unbundle(w409) -> ("Sample Period (s)"=w387:dbl, "Limits"=w393:T21, "Conditions"=w404:T25, "Overrides"=w381:T5, "Angular Limits"=w380:T6)
      n127 = Read from Binary File(5:w407, 8:w370, 11:w408) -> (0:w369:errorcluster, 2:w406:cluster{"x":dbl, "y":dbl, "th":dbl}[], 3:w398:refnum<file>)  [unwired: 3 in, 1 out]
      n128 = Read from Binary File(5:w405, 8:w369, 11:w398) -> (0:w368:errorcluster, 2:w383:cluster{"Time (s)":dbl, "Distance (ft)":dbl}, 3:w386:refnum<file>)  [unwired: 3 in, 1 out]
      n129 = Unbundle(w393) -> ("Velocity (fps)"=w391:dbl, "Accel (fps^2)"=w390:dbl, "Jerk (fps^3)"=w389:dbl, "StoopidFast (fps)"=w388:dbl)
      n130 = Bundle("Velocity (fps)"=w391, "Accel (fps^2)"=w390, "Jerk (fps^3)"=w389, "StoopidFast (fps)"=w388) -> (w392:T31)  [unwired: 1 in]
      n131 = Read from Binary File(5:FALSE, 8:w368, 11:w386) -> (0:w367:errorcluster, 2:w384:bool, 3:w379:refnum<file>)  [unwired: 3 in, 1 out]
      n132 = Read from Binary File(5:cluster{"Drive Type":T3, "Path Type":T4} {"Drive Type"=enum."Nonholonomic", "Path Type"=enum."Clothoid"} ("Trajectory Meta"), 11:w379) -> (2:w376:cluster{"Drive Type":T3, "Path Type":T4}, 3:w377:refnum<file>)  [unwired: 4 in, 2 out]
    }
  }
  "Zero V" <- w23
  "Reversals" <- w22
  "Commands out" <- w20
  "Points out" <- w18
  "Overall" <- w10
  "Trajectory Meta" <- w7
  "Trajectory Data" <- w4
  n133 = Bundle("Sample Period (s)"=w25, w26, "Conditions"=w27, "Overrides"=w28, "Angular Limits"=w8) -> (→"Fields":T7)  [unwired: 1 in]
  n134 = Close File(refnum=w15, error in=w1) -> (error out=→"error out":errorcluster)  [unwired: 1 out]
